vi "SetFrameRate.vi"(8 "error in (no error)":errorcluster, 10 "Frame Rate":u8, 11 "CameraTestingBL in":refnum<class "CameraTesting.lvclass">) -> (0 "error out":errorcluster, 3 "CameraTestingBL out":refnum<class "CameraTesting.lvclass">)   [LabVIEW 2020, in "CameraTesting.lvlib" / "CameraTesting.lvclass"]
doc: "Set the frame rate of the camera"
uses:
  CameraTesting.lvclass
  CameraTesting.lvclass/CameraTesting.ctl
  ICamera/ICamera/ICamera.lvclass
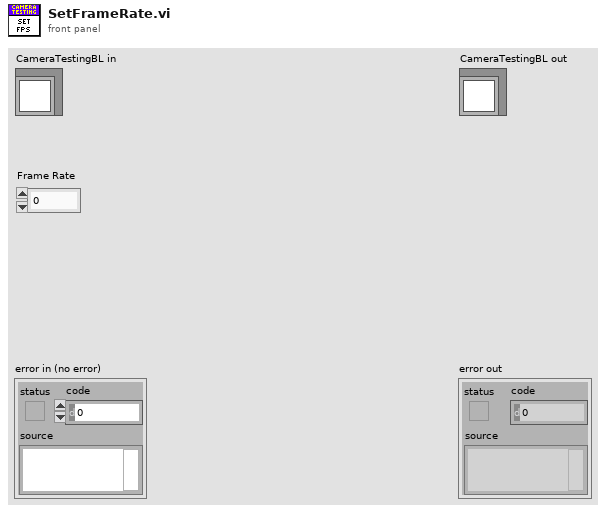
[diagram p1: front panel]
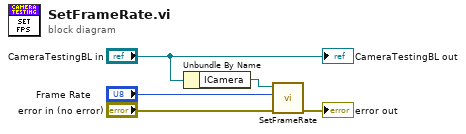
[diagram p0: block diagram]
diagram:
  n1 = Unbundle By Name("CameraTestingBL in") -> ("ICamera"=w5:refnum<class "ICamera.lvclass">)
  n2 = call-dynamic "SetFrameRate.vi"("error in (no error)"="error in (no error)", "Frame Rate (hex code)"="Frame Rate", "ICamera in"=w5) -> ("error out"=→"error out":errorcluster)  [unwired: 7 in, 1 out]
  "CameraTestingBL out" <- "CameraTestingBL in"
